vi "exnSharedSub read string as a variant type.vi"(5 "no change type":variant, 9 "type as string":string) -> (6 "type as variant":variant)   [LabVIEW 2017]
panel:
  in  "Boolean":bool
  in  "1D Array of Strings":string[](array[string])
  in  "String":string
  in  "1D Array of Waveforms":waveform(dbl)[](array[waveform])
  in  "Waveform":waveform(dbl)={"t0"=timestamp(0 s since 1904-01-01), "dt"=0.0, "Y"=[]}
  in  "DDT":dynamicdata(waveform)
  in  "2D Array of Numerics":dbl[][](array[numeric])
  in  "1D Array of Numerics":dbl[](array[numeric])
  in  "Numeric":dbl
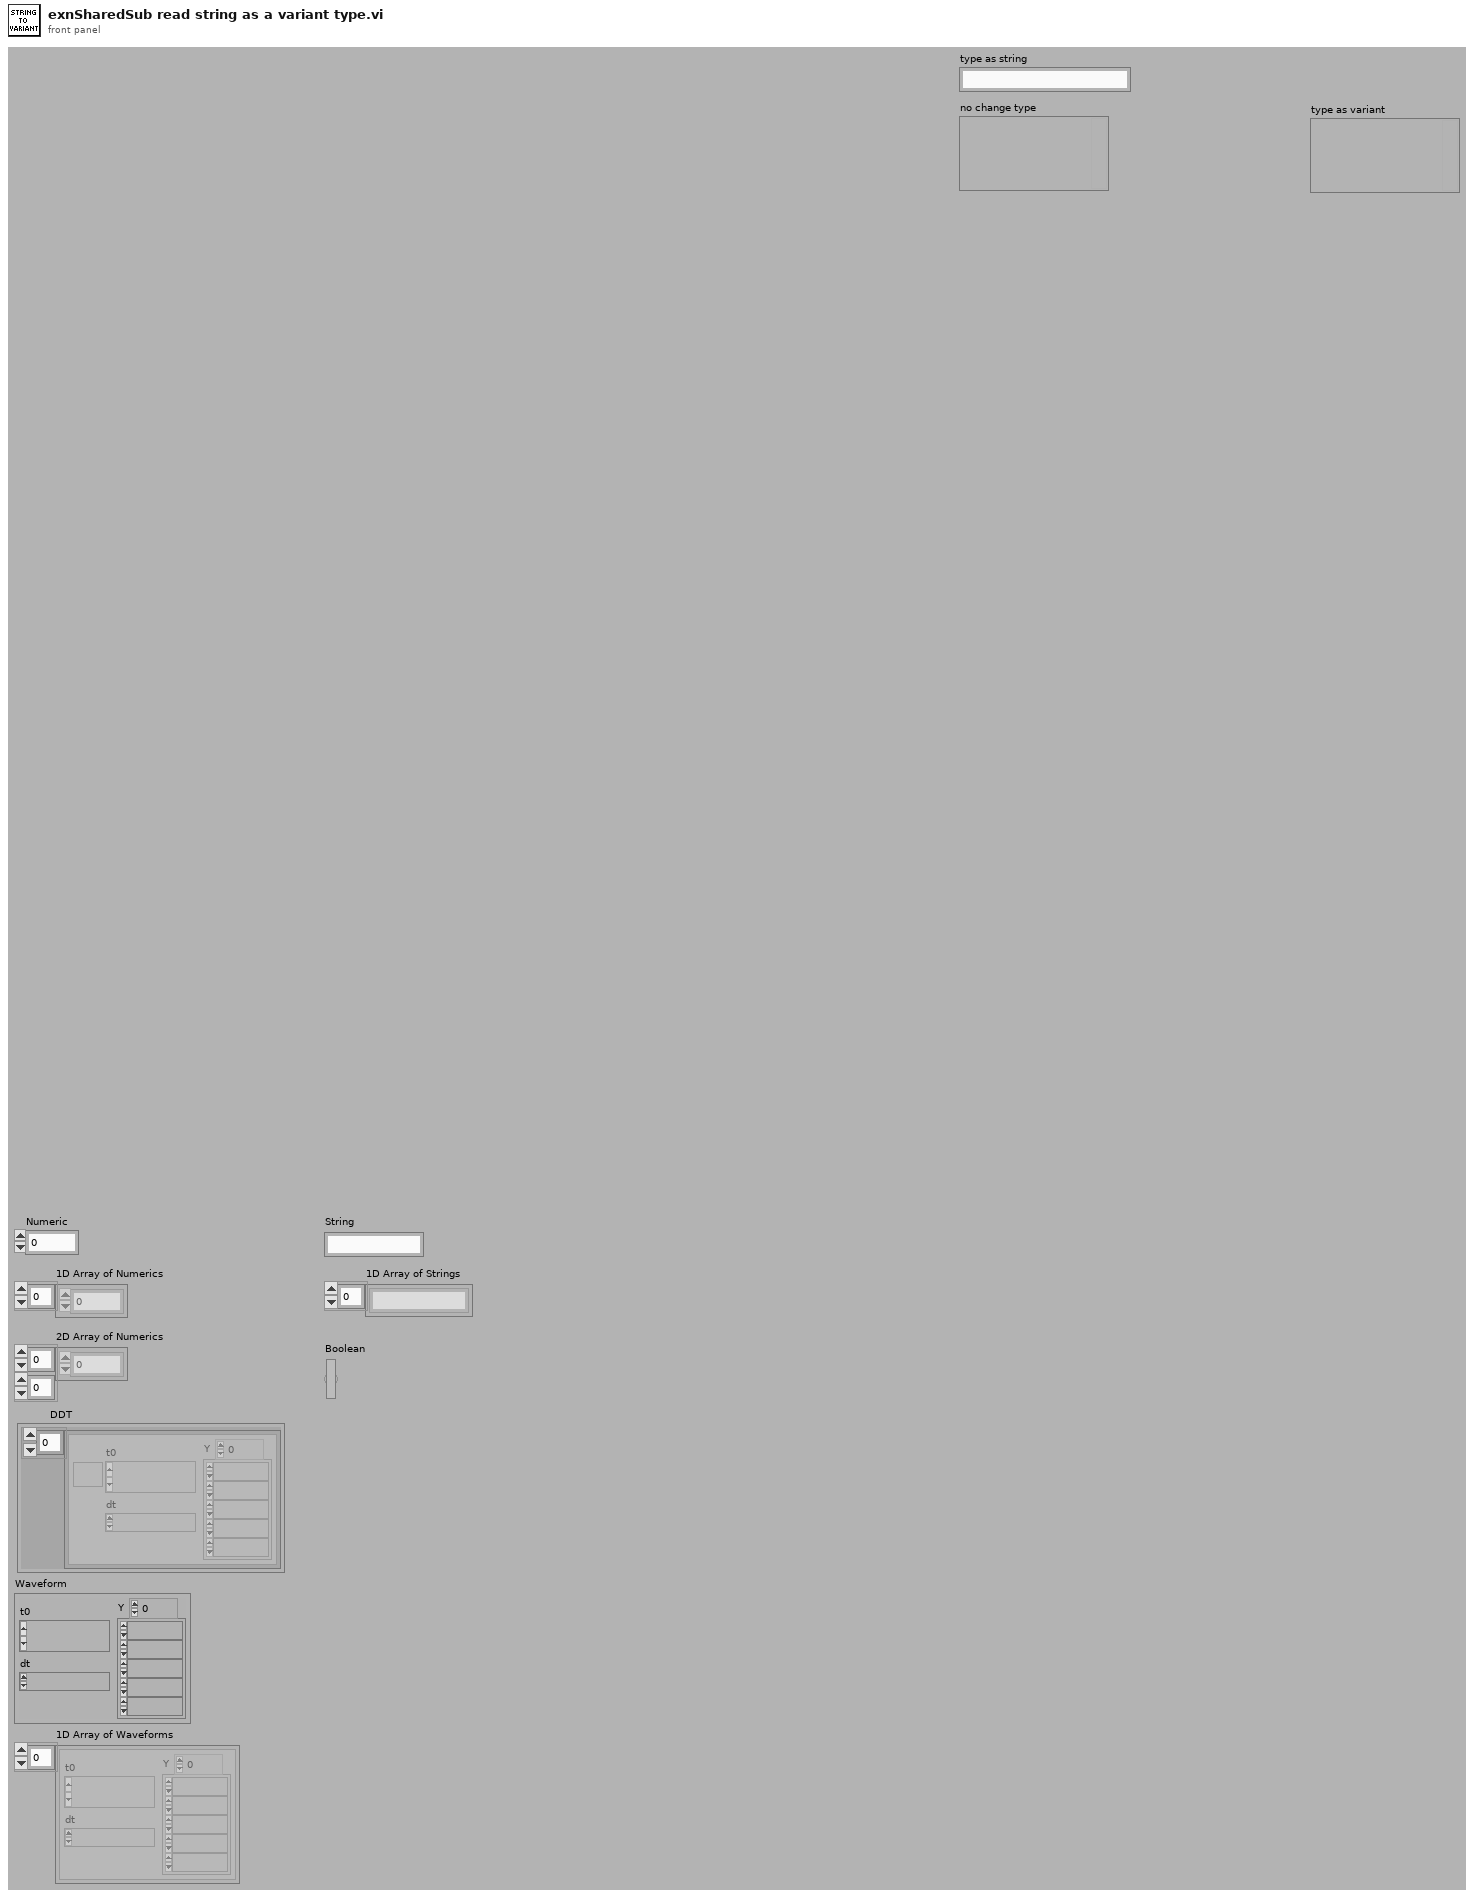
[diagram p1: front panel]
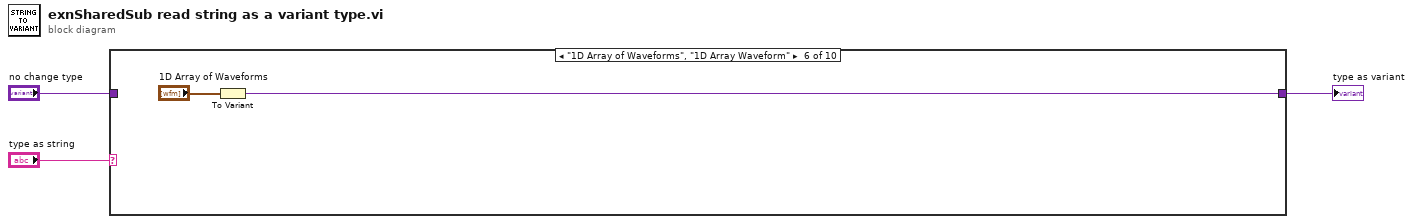
[diagram p0: block diagram]
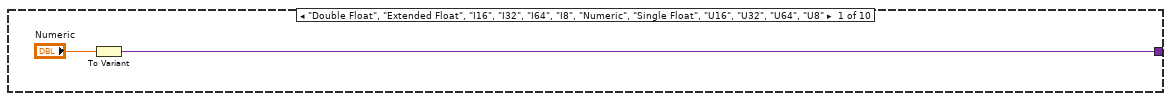
[diagram p2: hidden frame]
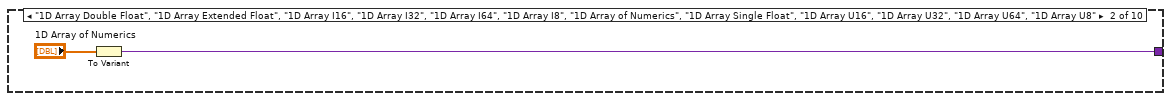
[diagram p3: hidden frame]
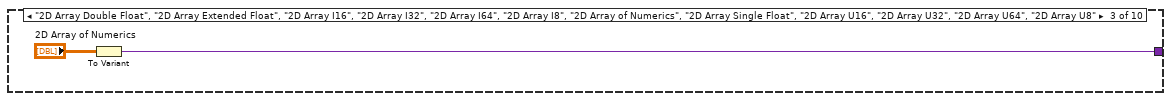
[diagram p4: hidden frame]
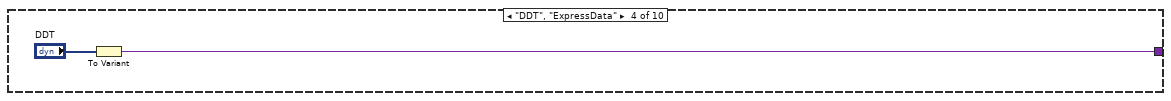
[diagram p5: hidden frame]
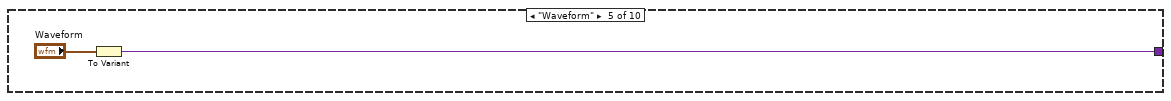
[diagram p6: hidden frame]
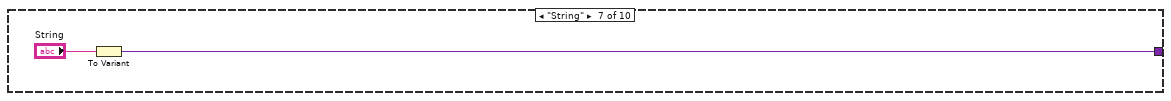
[diagram p7: hidden frame]
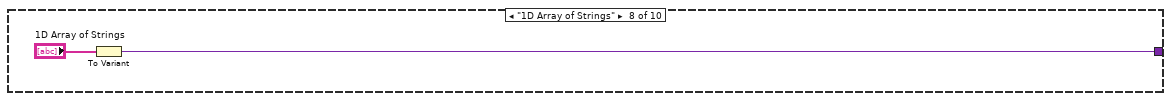
[diagram p8: hidden frame]
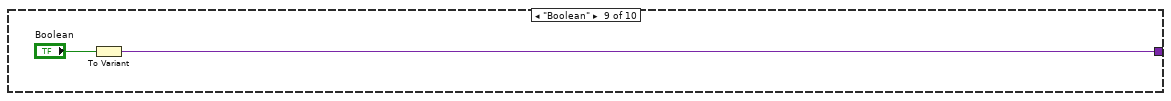
[diagram p9: hidden frame]
diagram:
  n1 = case shown="\"1D Array of Waveforms\", \"1D Array Waveform\"" "type as string" {
    tunnel: [w4 w7 w9 w11 w13 w15 w17 w19 w21 w22] -> w3
    tunnel: "no change type" -> [_ _ _ _ _ _ _ _ _ w22]
    frame "Double Float", "Extended Float", "I16", "I32", "I64", "I8", "Numeric", "Single Float", "U16", "U32", "U64", "U8" {
      n2 = To Variant(anything="Numeric") -> (Variant=w4:variant)
    }
    frame "1D Array Double Float", "1D Array Extended Float", "1D Array I16", "1D Array I32", "1D Array I64", "1D Array I8", "1D Array of Numerics", "1D Array Single Float", "1D Array U16", "1D Array U32", "1D Array U64", "1D Array U8" {
      n3 = To Variant(anything="1D Array of Numerics") -> (Variant=w7:variant)
    }
    frame "2D Array Double Float", "2D Array Extended Float", "2D Array I16", "2D Array I32", "2D Array I64", "2D Array I8", "2D Array of Numerics", "2D Array Single Float", "2D Array U16", "2D Array U32", "2D Array U64", "2D Array U8" {
      n4 = To Variant(anything="2D Array of Numerics") -> (Variant=w9:variant)
    }
    frame "DDT", "ExpressData" {
      n5 = To Variant(anything="DDT") -> (Variant=w11:variant)
    }
    frame "Waveform" {
      n6 = To Variant(anything="Waveform") -> (Variant=w13:variant)
    }
    frame "1D Array of Waveforms", "1D Array Waveform" {
      n7 = To Variant(anything="1D Array of Waveforms") -> (Variant=w15:variant)
    }
    frame "String" {
      n8 = To Variant(anything="String") -> (Variant=w17:variant)
    }
    frame "1D Array of Strings" {
      n9 = To Variant(anything="1D Array of Strings") -> (Variant=w19:variant)
    }
    frame "Boolean" {
      n10 = To Variant(anything="Boolean") -> (Variant=w21:variant)
    }
    frame "no change", Default {
    }
  }
  "type as variant" <- w3
